vi "OpenCreateReplace HDF5 File.vi"(4 "access_id":T1, 5 "create_id":T1, 6 "error in (no error)":errorcluster, 7 "function (open or create)":T2=enum."open or create", 9 "path":path) -> (0 "error out":errorcluster, 3 "HDF5 Ref out":T1)   [LabVIEW 2017]
doc: "Opens, creates, or replaces an HDF5 file."
uses:
  <vilib>/UPVI/lvhdf5/library.llb/HDF5 Ref.ctl
  <vilib>/UPVI/lvhdf5/file.llb/LVH5F Operation.ctl
  <vilib>/UPVI/lvhdf5/common.llb/To HDF5 Ref.vi
panel:
  # "LVHDF5 Toolkit\nCopyright (c) 2005-2013 by Jason D. Sommerville\nCopyright (c) 2014 by UPVI, LLC.\n\nThis use and distribution of this file is governed by the terms found in \nLICENSE.txt distributed with this toolkit and installed at\n <user.lib>\\_lvhdf5\\LICENSE.txt"
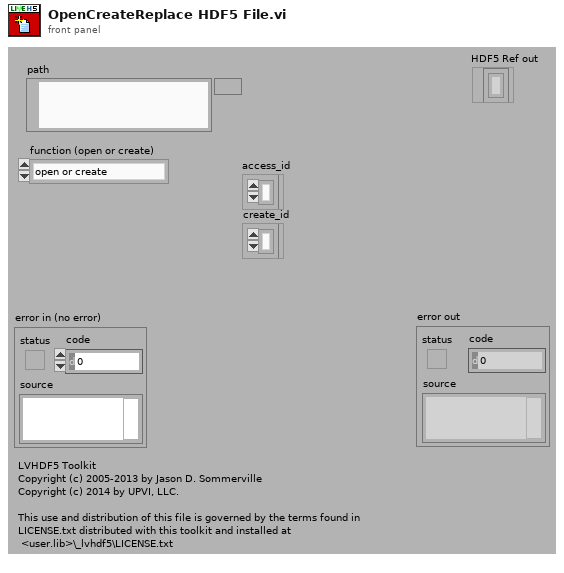
[diagram p1: front panel]
types:
  T1 = typedef "HDF5 Ref.ctl" = refnum<k1>
  T2 = typedef "LVH5F Operation.ctl" = enum16{"open", "open or create", "create or replace", "create or replace (with confirmation)", "create", "open (read only)"}
  T3 = enum16{"Left Button", "Center Button", "Right Button", "Window Close"}
  T4 = enum32{"existing file", "new file", "new or existing file", "existing dir", "new dir", "new or existing dir", "existing file (use LLBs)", "new file (use LLBs)", "new or existing file (use LLBs)", "new or existing file or directory (use LLBs)"}
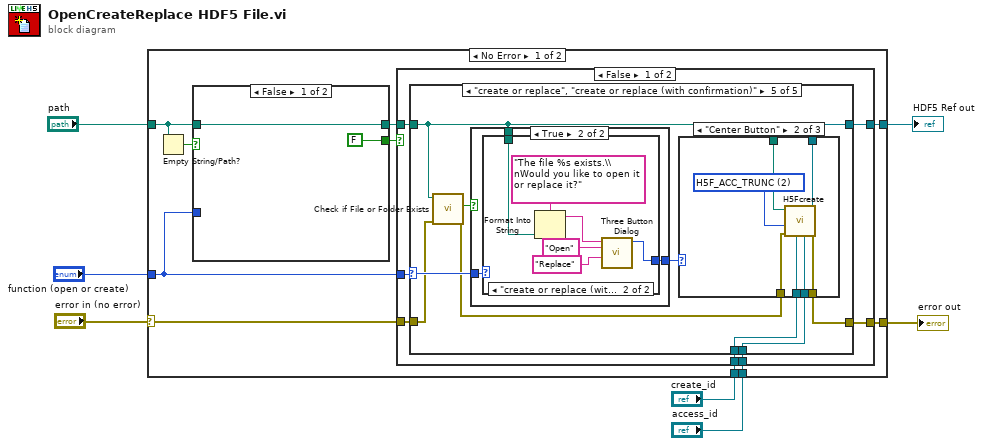
[diagram p0: block diagram]
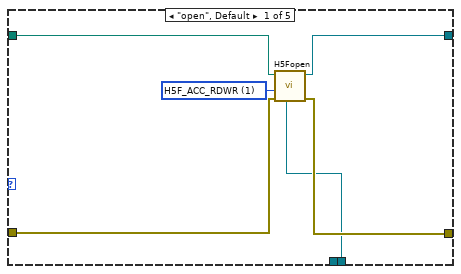
[diagram p2: hidden frame]
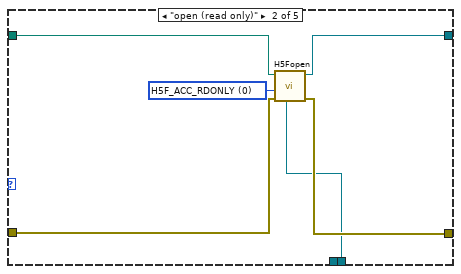
[diagram p3: hidden frame]
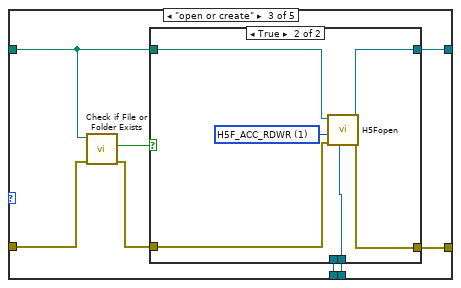
[diagram p4: hidden frame]
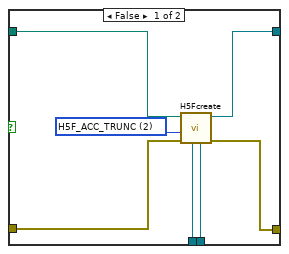
[diagram p5: hidden frame]
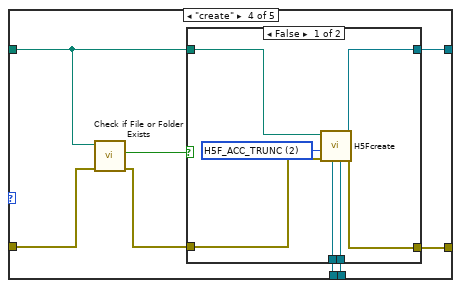
[diagram p6: hidden frame]
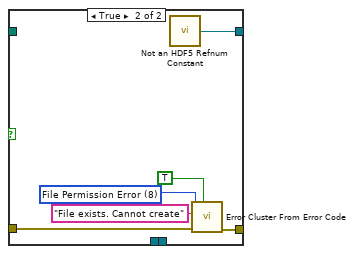
[diagram p7: hidden frame]
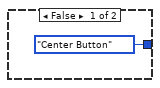
[diagram p8: hidden frame]
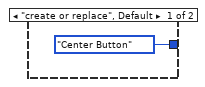
[diagram p9: hidden frame]
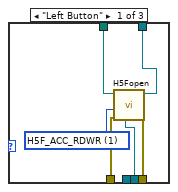
[diagram p10: hidden frame]
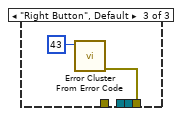
[diagram p11: hidden frame]
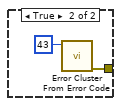
[diagram p12: hidden frame]
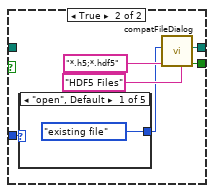
[diagram p13: hidden frame]
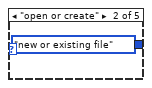
[diagram p14: hidden frame]
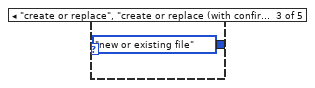
[diagram p15: hidden frame]
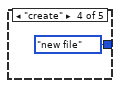
[diagram p16: hidden frame]
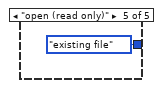
[diagram p17: hidden frame]
diagram:
  n1 = case shown="No Error" "error in (no error)" {
    selector: "error in (no error)" -> [w17 w130]
    tunnel: [w16 w130] -> w6
    tunnel: "function (open or create)" -> [w9 _]
    tunnel: "path" -> [w11 _]
    tunnel: [w15 _] -> w3
    tunnel: "access_id" -> [w14 _]
    tunnel: "create_id" -> [w13 _]
    frame No Error {
      n2 = Empty String/Path?(string/path=w11) -> (empty?=w12:bool)
      n3 = case shown="False" w12 {
        tunnel: w11 -> [w118 _]
        tunnel: [w118 w123] -> w10
        tunnel: w9 -> [_ w124]
        tunnel: [FALSE ("cancelled") w119] -> w8
        frame False {
        }
        frame True {
          n4 = case shown="\"open\", Default" w124 {
            tunnel: [T4."existing file" ("select mode (2)") T4."new or existing file" ("select mode (2)") T4."new or existing file" ("select mode (2)") T4."new file" ("select mode (2)") T4."existing file" ("select mode (2)")] -> w120
            frame "open", Default {
            }
            frame "open or create" {
            }
            frame "create or replace", "create or replace (with confirmation)" {
            }
            frame "create" {
            }
            frame "open (read only)" {
            }
          }
          n5 = call <vilib>:"compatFileDialog.vi"("pattern label"="HDF5 Files", "pattern"="*.h5;*.hdf5", "select mode (2)"=w120) -> ("cancelled"=w119:bool, "path"=w123:path)  [unwired: 6 in, 1 out]
        }
      }
      n6 = case shown="False" w8 {
        tunnel: w17 -> [w24 _]
        tunnel: [w23 w116] -> w16
        tunnel: [w22 _] -> w15
        tunnel: w14 -> [w21 _]
        tunnel: w13 -> [w20 _]
        tunnel: w10 -> [w19 _]
        tunnel: w9 -> [w18 _]
        frame False {
          n7 = case shown="\"create or replace\", \"create or replace (with confirmation)\"" w18 {
            selector: w18 -> [_ _ _ _ w84]
            tunnel: w24 -> [w29 w35 w38 w60 w82]
            tunnel: w19 -> [w28 w34 w40 w61 w81]
            tunnel: [w27 w33 w42 w63 w86] -> w23
            tunnel: [w26 w32 w44 w65 w88] -> w22
            tunnel: w21 -> [w25 w31 w43 w64 w87]
            tunnel: w20 -> [_ _ w41 w62 w85]
            frame "open", Default {
              w30 = u32 1 items=["H5F_ACC_RDONLY", "H5F_ACC_RDWR"] ("flags")
              n8 = call <vilib>:"H5Fopen.vi"("access_id"=w25, "error in (no error)"=w29, "flags"=w30, "path"=w28) -> ("error out"=w27:errorcluster, "HDF5 Ref out"=w26:T1)  [unwired: 4 in]
            }
            frame "open (read only)" {
              w36 = u32 0 items=["H5F_ACC_RDONLY", "H5F_ACC_RDWR"] ("flags")
              n9 = call <vilib>:"H5Fopen.vi"("access_id"=w31, "error in (no error)"=w35, "flags"=w36, "path"=w34) -> ("error out"=w33:errorcluster, "HDF5 Ref out"=w32:T1)  [unwired: 4 in]
            }
            frame "open or create" {
              n10 = call <vilib>:"Check if File or Folder Exists.vi"("error in (no error)"=w38, "path"=w40) -> ("error out"=w37:errorcluster, "file or folder exists?"=w39:bool)  [unwired: 7 in, 1 out]
              n11 = case shown="True" w39 {
                tunnel: w37 -> [w49 w56]
                tunnel: w40 -> [w46 w55]
                tunnel: [w45 w54] -> w44
                tunnel: w43 -> [w50 w53]
                tunnel: [w48 w52] -> w42
                tunnel: w41 -> [w51 _]
                frame False {
                  w47 = u32 2 items=["H5F_ACC_TRUNC"=2, "H5F_ACC_EXCL"=4] ("flags")
                  n12 = call <vilib>:"H5Fcreate.vi"("access_id"=w50, "create_id"=w51, "error in (no error)"=w49, "flags"=w47, "path"=w46) -> ("error out"=w48:errorcluster, "HDF5 Ref"=w45:T1)  [unwired: 3 in]
                }
                frame True {
                  w57 = u32 1 items=["H5F_ACC_RDONLY", "H5F_ACC_RDWR"] ("flags")
                  n13 = call <vilib>:"H5Fopen.vi"("access_id"=w53, "error in (no error)"=w56, "flags"=w57, "path"=w55) -> ("error out"=w52:errorcluster, "HDF5 Ref out"=w54:T1)  [unwired: 4 in]
                }
              }
            }
            frame "create" {
              n14 = call <vilib>:"Check if File or Folder Exists.vi"("error in (no error)"=w60, "path"=w61) -> ("error out"=w59:errorcluster, "file or folder exists?"=w58:bool)  [unwired: 7 in, 1 out]
              n15 = case shown="False" w58 {
                tunnel: w59 -> [w70 w77]
                tunnel: w61 -> [w67 _]
                tunnel: [w66 w73] -> w65
                tunnel: w64 -> [w71 _]
                tunnel: [w69 w78] -> w63
                tunnel: w62 -> [w72 _]
                frame False {
                  w68 = u32 2 items=["H5F_ACC_TRUNC"=2, "H5F_ACC_EXCL"=4] ("flags")
                  n16 = call <vilib>:"H5Fcreate.vi"("access_id"=w71, "create_id"=w72, "error in (no error)"=w70, "flags"=w68, "path"=w67) -> ("error out"=w69:errorcluster, "HDF5 Ref"=w66:T1)  [unwired: 3 in]
                }
                frame True {
                  w75 = u16 8 items=["No Error", "Argument Error", "Memory Full", "Out of Zone", "End of File", "File Already Open", "Generic File IO Error", "File Not Found", "File Permission Error", "Disk Full", "Duplicate Path", "Too Many Files Open", "Not Enabled", "Resource File Not Found", "Cannot Add Resource", "Resource Not Found", "Image Not Found", "Image Memory Error", "Pen Does Not Exist", "Config Bad Type", "Config Token Not Found", "Config Parse Error", "Config Memory Error", "Bad External Code Format", "Bad External Code Offset", "External Code Not Present", "Null Window", "Destroy Window Mixup", "Null Menu", "Print Aborted", "Bad Print Record", "Print Driver Error", "Windows Error During Print", "Memory Error During Print", "Print Dialog Error", "Generic Print Error", "Invalid Device Refnum", "Device Not Found", "Device Parameter Error", "Device Unit Error", "Can't Open Device", "Device Call Aborted", "Generic Error", "Cancelled By User", "Object ID Too Low", "Object ID Too High", "Object Not In Heap", "Unknown Heap", "Bad DefProc ID", "DefProc Not In Table", "Message Out Of Range", "Null Method", "Unknown Message", "Manager Call Not Supported", "Bad address", "Connection In progress", "Connection timed out", "Connection is already in progress", "Network attribute not supported", "Network error", "Address in use", "System out of memory", "Connection aborted", "Connection refused", "Connection is not connected", "Connection is already connected", "Connection closed", "Initialize error (interapplication manager)", "Bad occurrence", "Wait on unbound occurrence handler", "Occurrence queue overflow", "Bad path", "Semaphore not signaled", "Unrecognized type (interapplication manager)"]
                  n17 = call <vilib>:"Not an HDF5 Refnum Constant.vi"() -> ("HDF5 Ref"=w73:T1)
                  n18 = call <vilib>:"Error Cluster From Error Code.vi"("show call chain? (False)"=TRUE, "error in (no error)"=w77, "error message (\"\")"="File exists. Cannot create" ("error message (\"\")"), "error code (0)"=w75) -> ("error out"=w78:errorcluster)  [unwired: 5 in]
                }
              }
            }
            frame "create or replace", "create or replace (with confirmation)" {
              n19 = call <vilib>:"Check if File or Folder Exists.vi"("error in (no error)"=w82, "path"=w81) -> ("error out"=w80:errorcluster, "file or folder exists?"=w79:bool)  [unwired: 7 in, 1 out]
              n20 = case shown="True" w79 {
                tunnel: w84 -> [_ w92]
                tunnel: [T3."Center Button" ("Which Button?") w91] -> w83
                tunnel: w81 -> [_ w90]
                frame False {
                }
                frame True {
                  n21 = case shown="\"create or replace (with confirmation)\"" w92 {
                    tunnel: w90 -> [_ w98]
                    tunnel: [T3."Center Button" ("Which Button?") w94] -> w91
                    frame "create or replace", Default {
                    }
                    frame "create or replace (with confirmation)" {
                      n22 = Format Into String(format string="The file %s exists.\\nWould you like to open it or replace it?", w98) -> (resulting string=w97:string)  [unwired: 2 in, 1 out]
                      n23 = call <vilib>:"Three Button Dialog.vi"("Center Button Text (\"No\")"="Replace" ("Center Button Text (\"No\")"), "Left Button Text (\"Yes\")"="Open" ("Left Button Text (\"Yes\")"), "message"=w97) -> ("Which Button?"=w94:T3)  [unwired: 8 in]
                    }
                  }
                }
              }
              n24 = case shown="\"Center Button\"" w83 {
                tunnel: w80 -> [w104 w112 _]
                tunnel: w81 -> [w101 w111 _]
                tunnel: [w100 w110 _] -> w88
                tunnel: w87 -> [w102 w109 _]
                tunnel: [w103 w108 w113] -> w86
                tunnel: w85 -> [_ w107 _]
                frame "Left Button" {
                  w105 = u32 1 items=["H5F_ACC_RDONLY", "H5F_ACC_RDWR"] ("flags")
                  n25 = call <vilib>:"H5Fopen.vi"("access_id"=w102, "error in (no error)"=w104, "flags"=w105, "path"=w101) -> ("error out"=w103:errorcluster, "HDF5 Ref out"=w100:T1)  [unwired: 4 in]
                }
                frame "Center Button" {
                  w106 = u32 2 items=["H5F_ACC_TRUNC"=2, "H5F_ACC_EXCL"=4] ("flags")
                  n26 = call <vilib>:"H5Fcreate.vi"("access_id"=w109, "create_id"=w107, "error in (no error)"=w112, "flags"=w106, "path"=w111) -> ("error out"=w108:errorcluster, "HDF5 Ref"=w110:T1)  [unwired: 3 in]
                }
                frame "Right Button", Default {
                  n27 = call <vilib>:"Error Cluster From Error Code.vi"("error code (0)"=43) -> ("error out"=w113:errorcluster)  [unwired: 8 in]
                }
              }
            }
          }
        }
        frame True {
          n28 = call <vilib>:"Error Cluster From Error Code.vi"("error code (0)"=43) -> ("error out"=w116:errorcluster)  [unwired: 8 in]
        }
      }
    }
    frame Error {
    }
  }
  "error out" <- w6
  "HDF5 Ref out" <- w3
